vi "Sensor Locations.vi"(10 "Ref Array":refnum<vi>[](array[refnum]), 11 "Data Cluster In":T1={"Selected File"=path "", "Full Text File"=[], "Data Array"=[], "Times Array"=[], "Sensor Array"=[], "Subset Array"=[], "Smoothness Values"=[], "Sensor Select 1"=refnum, "Sensor Select 2"=refnum, "Sensor Select 3"=refnum, "Sensor Select 4"=refnum, "Start Times"=[], "End Times"=[], "Cursor List"=[{"Name"="Event Marker          ", "Color"=16777200, "Style"=0, "Point Style"=0, "Name Visible"=FALSE, "Allow Drag"=FALSE, "Cursor Mode"=0, "Plot"=0, "Index"=0, "Position"={"X"=4.0, "Y"=1.0}, "X Scale"=0, "Y Scale"=0, "Watch Plots"=[], "Watch All Plots"=FALSE, "Plot Area"=0, "Label Offset"={"X"=-50.0, "Y"=150.0}}, {"Name"="Upper Sensor", "Color"=13816500, "Style"=6, "Point Style"=0, "Name Visible"=FALSE, "Allow Drag"=FALSE, "Cursor Mode"=0, "Plot"=0, "Index"=0, "Position"={"X"=-1.0, "Y"=5.0}, "X Scale"=0, "Y Scale"=0, "Watch Plots"=[], "Watch All Plots"=FALSE, "Plot Area"=0, "Label Offset"={"X"=0.0, "Y"=0.0}}, {"Name"="Lower Sensor", "Color"=13816500, "Style"=6, "Point Style"=0, "Name Visible"=FALSE, "Allow Drag"=FALSE, "Cursor Mode"=0, "Plot"=0, "Index"=0, "Position"={"X"=-1.0, "Y"=30.0}, "X Scale"=0, "Y Scale"=0, "Watch Plots"=[], "Watch All Plots"=FALSE, "Plot Area"=0, "Label Offset"={"X"=0.0, "Y"=0.0}}], "Listbox 1"=refnum, "Listbox 2"=refnum, "Listbox 3"=refnum, "Listbox 4"=refnum, "Labels"=["Why", "is", "this", "still", "not", "built", "into", "Labview?", "This", "is", "shameful."], "Event Array"=[], "Event Names"=[], "Event Times"=[], "Save Plot Button"=refnum, "Sensor Plot Refs"=[], "Selected Event (Title)"="", "Upper Cursor"=0.0, "Lower Cursor"=0.0, "Z Max"=0.0, "Z Min"=0.0}) -> (2 "Sensors":string, 3 "Locations":string)   [LabVIEW 2021]
uses:
  Controls/DataCluster.ctl
  <vilib>/Utility/miscctls.llb/LVCursorListTypeDef.ctl
  <vilib>/express/express shared/transition.llb/Dynamic To Waveform Array.vi
  <vilib>/express/express signal manip/GetorSetDDTAttributes/Get DDT Attributes/Get DDT Properties.xnode
panel:
  out "Array":string[][](array[string])
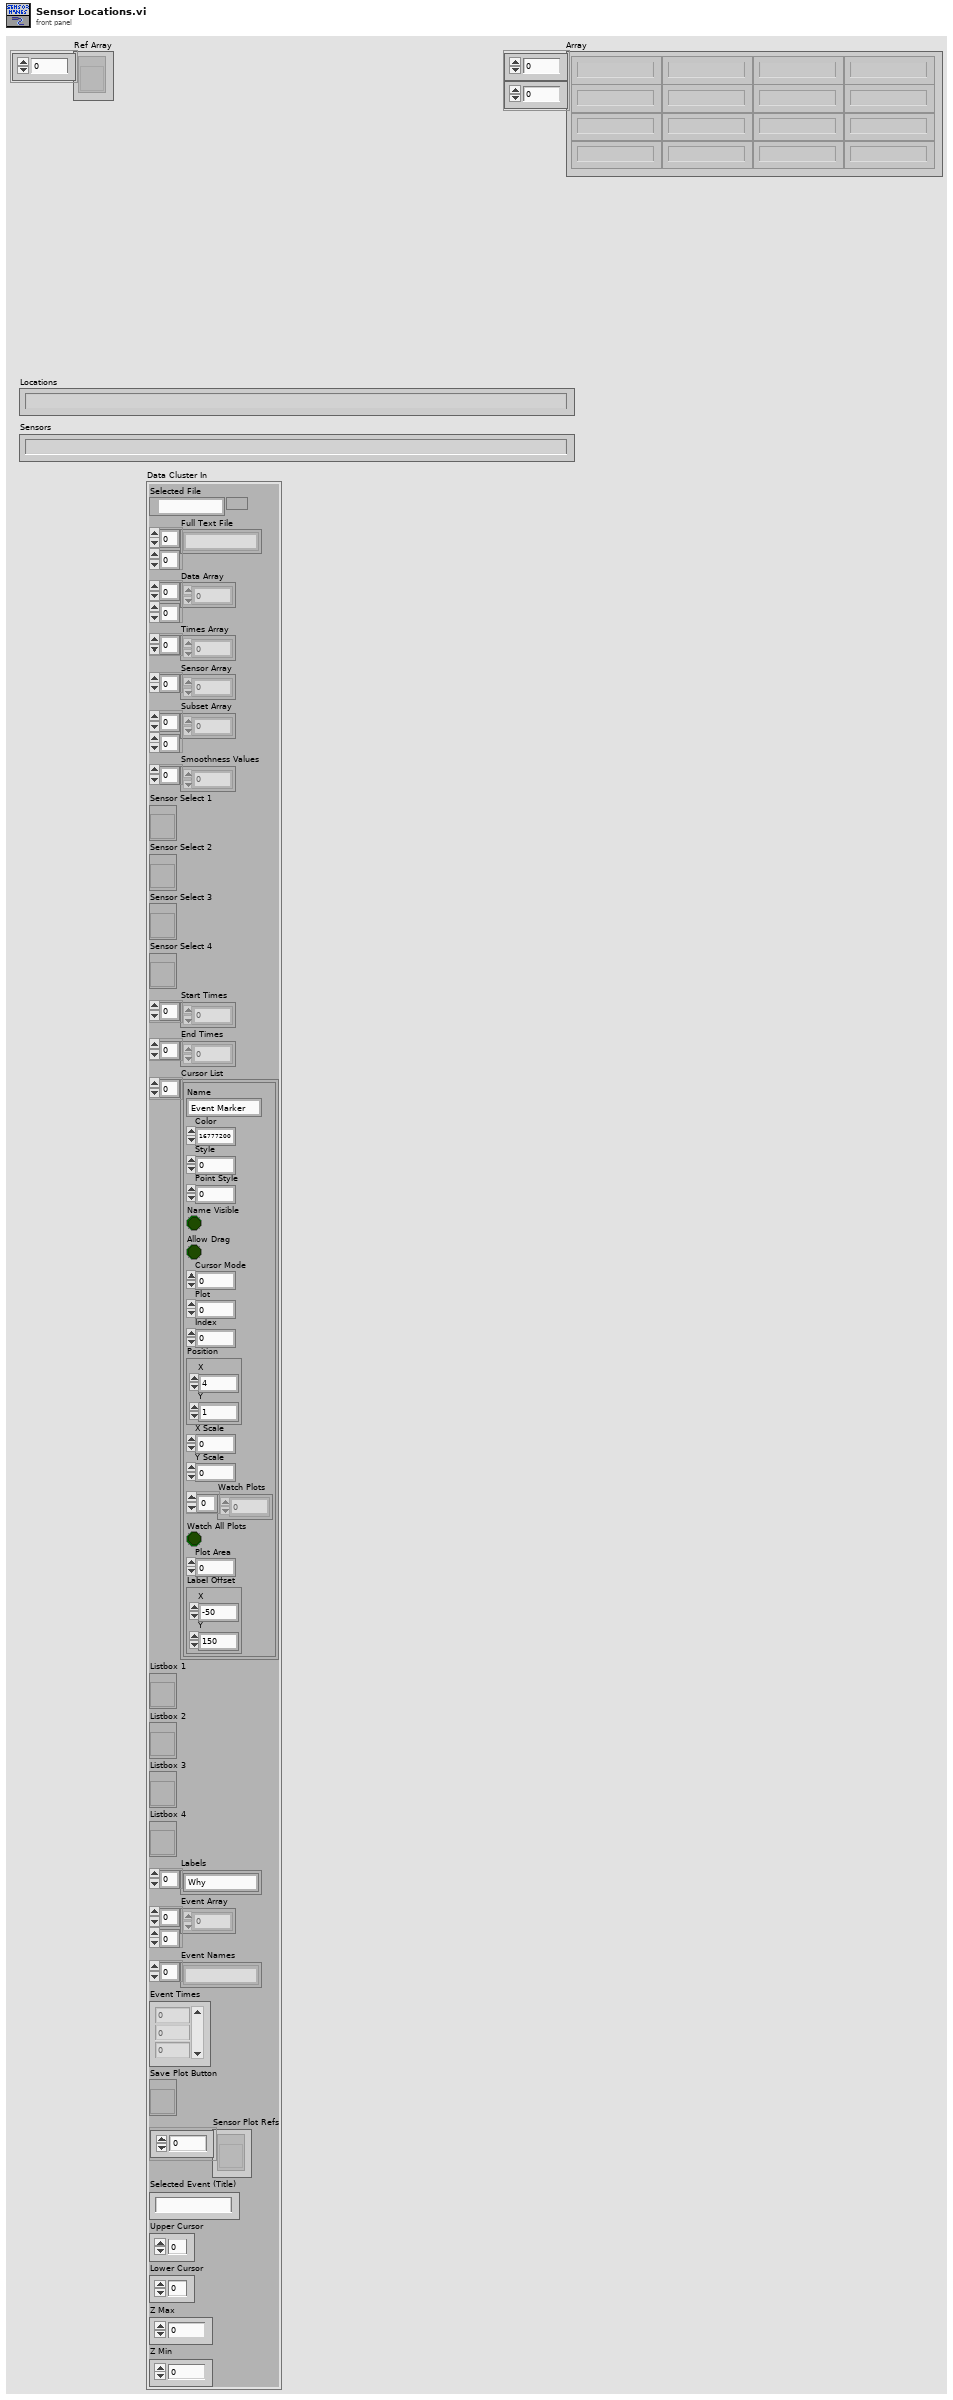
[diagram p1: front panel]
types:
  T1 = typedef "DataCluster.ctl" = cluster{"Selected File":path, "Full Text File":string[][], "Data Array":dbl[][], "Times Array":dbl[], "Sensor Array":dbl[], "Subset Array":dbl[][], "Smoothness Values":dbl[], "Sensor Select 1":refnum<vi>, "Sensor Select 2":refnum<vi>, "Sensor Select 3":refnum<vi>, "Sensor Select 4":refnum<vi>, "Start Times":dbl[], "End Times":dbl[], "Cursor List":T2, "Listbox 1":refnum<vi>, "Listbox 2":refnum<vi>, "Listbox 3":refnum<vi>, "Listbox 4":refnum<vi>, "Labels":string[], "Event Array":dbl[][], "Event Names":string[], "Event Times":dbl[], "Save Plot Button":refnum<vi>, "Sensor Plot Refs":refnum<vi>[], "Selected Event (Title)":string, "Upper Cursor":dbl, "Lower Cursor":dbl, "Z Max":dbl, "Z Min":dbl}
  T2 = typedef "LVCursorListTypeDef.ctl" = cluster{"Name":string, "Color":u32, "Style":u8, "Point Style":u8, "Name Visible":bool, "Allow Drag":bool, "Cursor Mode":u32, "Plot":i32, "Index":i32, "Position":cluster{"X":dbl, "Y":dbl}, "X Scale":u32, "Y Scale":u32, "Watch Plots":i32[], "Watch All Plots":bool, "Plot Area":i32, "Label Offset":cluster{"X":dbl, "Y":dbl}}[]
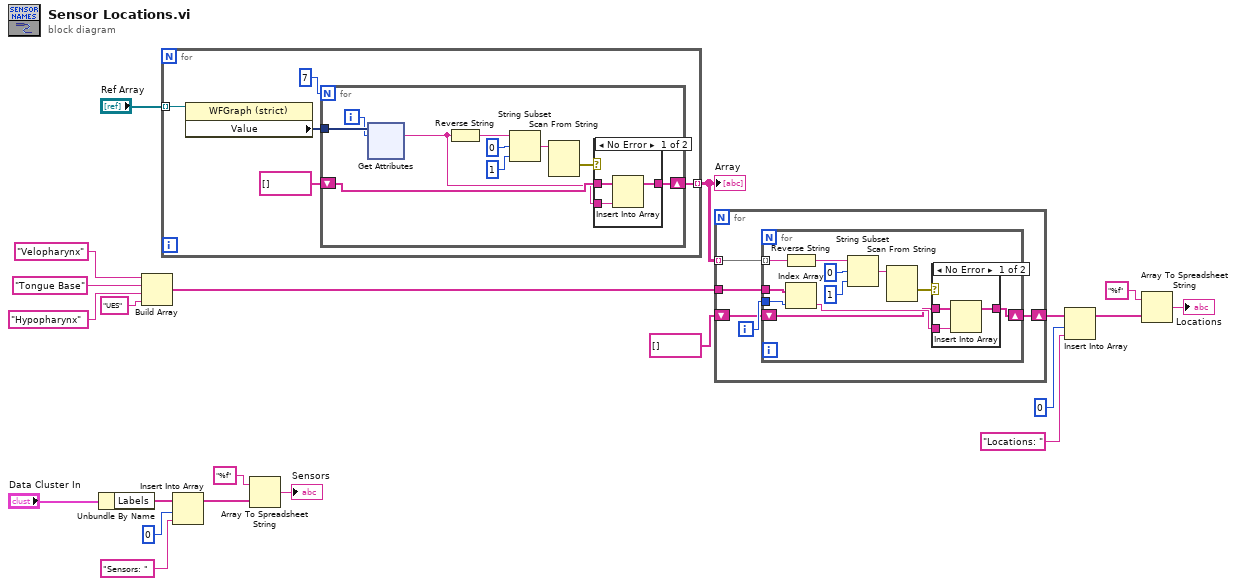
[diagram p0: block diagram]
diagram:
  n1 = Unbundle By Name("Data Cluster In") -> ("Labels"=w2:string[])
  n2 = Build Array("Velopharynx", "Tongue Base", "Hypopharynx", "UES") -> (w5:string[])
  n3 = for {
    tunnel: "Ref Array" -> [w26] mode=indexing
    tunnel: [w22] -> w10 mode=indexing
    n4 = property class="WFGraph (strict)"(reference=w26) -> ("Value"=w24:dynamicdata)  [unwired: 1 in, 2 out]
    n5 = for {
      N: 7 -> [_]
      shift-right: [w35] -> w22
      shift-left: string[] [] -> [w36]
      tunnel: w24 -> [w29]
      i -> [w28]
      n6 = xnode "Get Attributes"("Signals In"=w29, "Signal Index"=w28) -> ("Signal Name"=w27:string)  [unwired: 1 in, 2 out]
      n7 = Reverse String(1:w27) -> (0:w33:string)
      n8 = String Subset(string=w33, offset (0)=0, length (rest)=1 ("length (rest)")) -> (substring=w31:string)
      n9 = Scan From String(input string=w31) -> (error out=w30:errorcluster)  [unwired: 5 in, 2 out]
      n10 = case shown="No Error" w30 {
        tunnel: w36 -> [w48 w49]
        tunnel: [w47 w49] -> w35
        tunnel: w27 -> [w46 _]
        frame No Error {
          n11 = Insert Into Array(array=w48, new element=w46) -> (w47:string[])  [unwired: 1 in]
        }
        frame Error {
        }
      }
    }
  }
  "Array" <- w10
  n12 = Insert Into Array(array=w2, index=0, new element="Sensors: " ("new element/subarray")) -> (w13:string[])
  n13 = Array To Spreadsheet String(array=w13, 3:"%f" ("format string")) -> (spreadsheet string=→"Sensors":string)  [unwired: 1 in]
  n14 = for {
    tunnel: w10 -> [w54] mode=indexing
    tunnel: w5 -> [w53]
    shift-right: [w50] -> w3
    shift-left: string[] [] -> [w51]
    i -> [w52]
    n15 = for {
      tunnel: w54 -> [w58] mode=indexing
      tunnel: w53 -> [w65]
      tunnel: w52 -> [w64]
      shift-right: [w56] -> w50
      shift-left: w51 -> [w57]
      n16 = Reverse String(1:w58) -> (0:w63:string)
      n17 = Index Array(array=w65, index=w64) -> (element=w59:string)
      n18 = String Subset(string=w63, offset (0)=0, length (rest)=1 ("length (rest)")) -> (substring=w61:string)
      n19 = Scan From String(input string=w61) -> (error out=w60:errorcluster)  [unwired: 5 in, 2 out]
      n20 = case shown="No Error" w60 {
        tunnel: w57 -> [w68 w69]
        tunnel: [w67 w69] -> w56
        tunnel: w59 -> [w66 _]
        frame No Error {
          n21 = Insert Into Array(array=w68, new element=w66) -> (w67:string[])  [unwired: 1 in]
        }
        frame Error {
        }
      }
    }
  }
  n22 = Insert Into Array(array=w3, index=0, new element="Locations: " ("new element/subarray")) -> (w17:string[])
  n23 = Array To Spreadsheet String(array=w17, 3:"%f" ("format string")) -> (spreadsheet string=→"Locations":string)  [unwired: 1 in]
